vi "Write Observation.vi"(8 "error in (no error)":errorcluster, 10 "Observer":refnum<class "Send.lvclass">, 11 "ObserverRegistryCommand.lvclass in":refnum<class "ObserverRegistryCommand.lvclass">) -> (0 "error out":errorcluster, 3 "ObserverRegistryCommand.lvclass out":refnum<class "ObserverRegistryCommand.lvclass">)   [LabVIEW 2011, in "Messenging.lvlib" / "ObserverRegistryCommand.lvclass"]
uses:
  ObserverRegistryCommand.lvclass
  Interprocess Messenger/Send/Send.lvclass
  ObserverRegistryCommand.lvclass/ObserverRegistryCommand.ctl
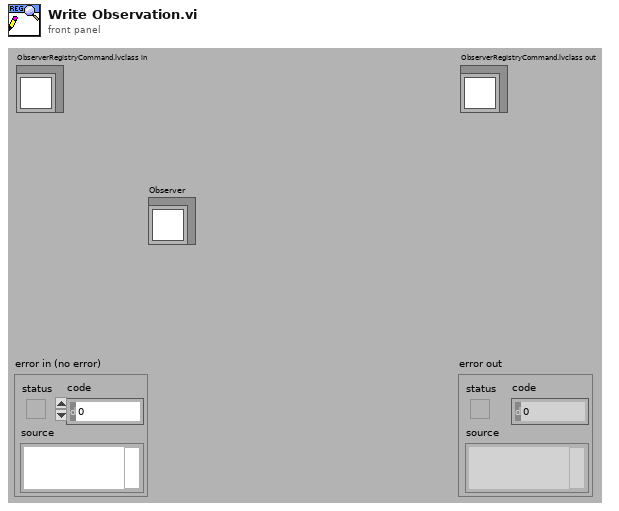
[diagram p1: front panel]
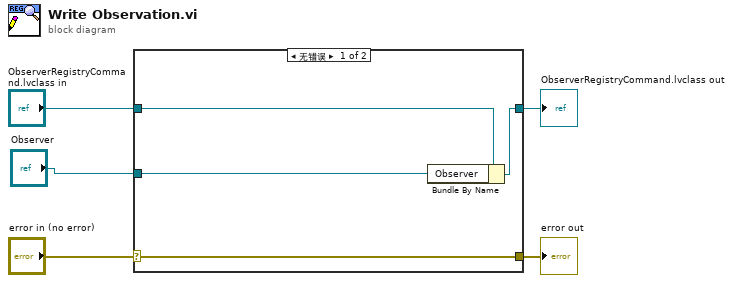
[diagram p0: block diagram]
diagram:
  n1 = case shown="无错误" "error in (no error)" {
    selector: "error in (no error)" -> [w9 w10]
    tunnel: [w9 w10] -> w4
    tunnel: [w7 w11] -> w2
    tunnel: "ObserverRegistryCommand.lvclass in" -> [w8 w11]
    tunnel: "Observer" -> [w6 _]
    frame No Error {
      n2 = Bundle By Name(cluster=w8, "Observer"=w6) -> (w7:refnum<class "ObserverRegistryCommand.lvclass">)
    }
    frame Error {
    }
  }
  "error out" <- w4
  "ObserverRegistryCommand.lvclass out" <- w2
